vi "from string 2.0.vi"(8 "error in (no error)":errorcluster, 10 "data":string, 11 "PID Module configuration in":refnum<class "PID Module configuration.lvclass">) -> (0 "error out":errorcluster, 3 "PID Module configuration out":refnum<class "PID Module configuration.lvclass">)   [LabVIEW 2015, in "PID Module configuration.lvclass"]
uses:
  PID Module configuration.lvclass
  <vilib>/NI/Tag Bus Module Framework/channel/TBM channel.lvclass
  Line.ctl
  PID Module configuration.lvclass/PID Module configuration.ctl
  <vilib>/NI/Configuration Framework/serializable configuration/NISE_CEF_serializable configuration.lvclass
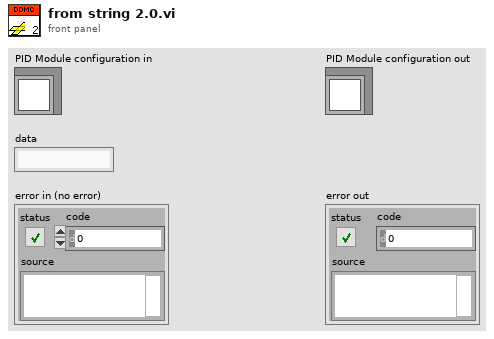
[diagram p1: front panel]
types:
  T1 = typedef "PID Module configuration.lvclass/Line.ctl" = cluster{"PID ID":string, "Setpoint":refnum<class "TBM channel.lvclass">, "Variable":refnum<class "TBM channel.lvclass">, "Output":refnum<class "TBM channel.lvclass">, "Output High":refnum<class "TBM channel.lvclass">, "Output Low":refnum<class "TBM channel.lvclass">, "P":refnum<class "TBM channel.lvclass">, "I":refnum<class "TBM channel.lvclass">, "D":refnum<class "TBM channel.lvclass">}
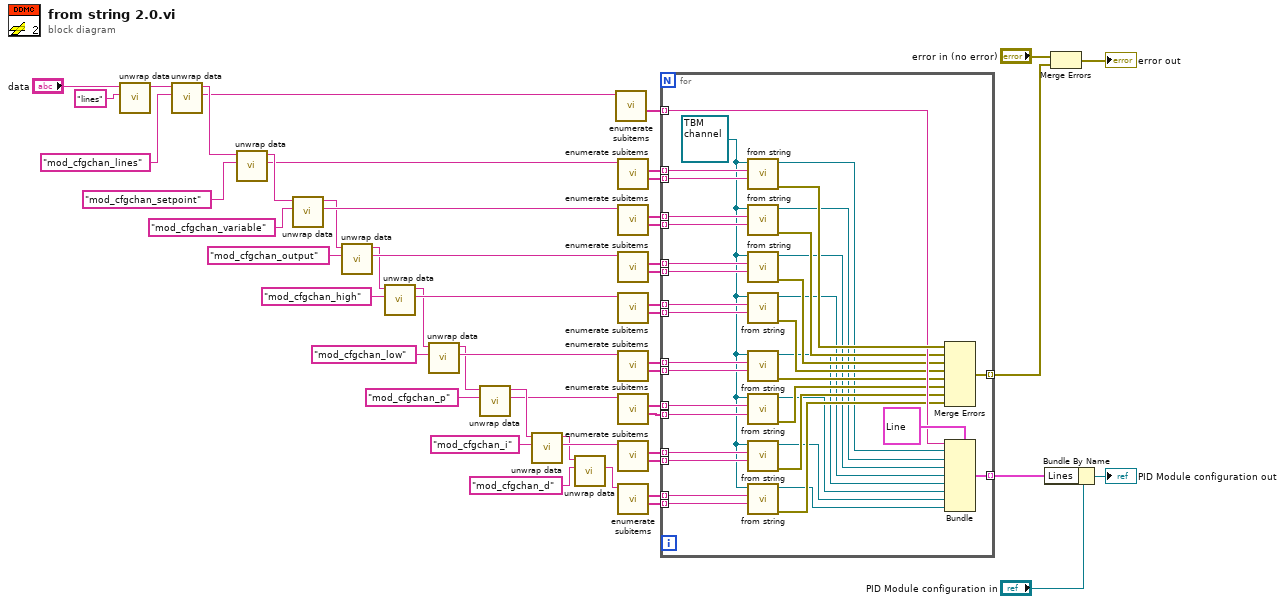
[diagram p0: block diagram]
diagram:
  n1 = call <vilib>:"unwrap data.vi"("identifier"="lines" ("additional identifier"), "data to unwrap"="data") -> ("remaining string"=w49:string)  [unwired: 8 in, 1 out]
  n2 = call <vilib>:"unwrap data.vi"("identifier"="mod_cfgchan_lines", "data to unwrap"=w49) -> ("unwrapped data"=w18:string, "remaining string"=w37:string)  [unwired: 8 in]
  n3 = call <vilib>:"unwrap data.vi"("identifier"="mod_cfgchan_setpoint", "data to unwrap"=w37) -> ("unwrapped data"=w17:string, "remaining string"=w36:string)  [unwired: 8 in]
  n4 = call <vilib>:"unwrap data.vi"("identifier"="mod_cfgchan_variable", "data to unwrap"=w36) -> ("unwrapped data"=w44:string, "remaining string"=w35:string)  [unwired: 8 in]
  n5 = call <vilib>:"unwrap data.vi"("identifier"="mod_cfgchan_output", "data to unwrap"=w35) -> ("unwrapped data"=w43:string, "remaining string"=w34:string)  [unwired: 8 in]
  n6 = call <vilib>:"unwrap data.vi"("identifier"="mod_cfgchan_high", "data to unwrap"=w34) -> ("unwrapped data"=w42:string, "remaining string"=w33:string)  [unwired: 8 in]
  n7 = call <vilib>:"unwrap data.vi"("identifier"="mod_cfgchan_low", "data to unwrap"=w33) -> ("unwrapped data"=w41:string, "remaining string"=w32:string)  [unwired: 8 in]
  n8 = call <vilib>:"unwrap data.vi"("identifier"="mod_cfgchan_p", "data to unwrap"=w32) -> ("unwrapped data"=w22:string, "remaining string"=w31:string)  [unwired: 8 in]
  n9 = call <vilib>:"unwrap data.vi"("identifier"="mod_cfgchan_i", "data to unwrap"=w31) -> ("unwrapped data"=w40:string, "remaining string"=w30:string)  [unwired: 8 in]
  n10 = call <vilib>:"unwrap data.vi"("identifier"="mod_cfgchan_d", "data to unwrap"=w30) -> ("unwrapped data"=w21:string)  [unwired: 8 in, 1 out]
  n11 = call <vilib>:"enumerate subitems.vi"("data to enumerate"=w18) -> ("associated data"=w16:string[])  [unwired: 8 in, 2 out]
  n12 = call <vilib>:"enumerate subitems.vi"("data to enumerate"=w17) -> ("associated data"=w51:string[], "discovered subitems"=w50:string[])  [unwired: 8 in, 1 out]
  n13 = call <vilib>:"enumerate subitems.vi"("data to enumerate"=w44) -> ("associated data"=w14:string[], "discovered subitems"=w15:string[])  [unwired: 8 in, 1 out]
  n14 = call <vilib>:"enumerate subitems.vi"("data to enumerate"=w43) -> ("associated data"=w12:string[], "discovered subitems"=w13:string[])  [unwired: 8 in, 1 out]
  n15 = call <vilib>:"enumerate subitems.vi"("data to enumerate"=w42) -> ("associated data"=w10:string[], "discovered subitems"=w11:string[])  [unwired: 8 in, 1 out]
  n16 = call <vilib>:"enumerate subitems.vi"("data to enumerate"=w41) -> ("associated data"=w8:string[], "discovered subitems"=w9:string[])  [unwired: 8 in, 1 out]
  n17 = call <vilib>:"enumerate subitems.vi"("data to enumerate"=w22) -> ("associated data"=w6:string[], "discovered subitems"=w7:string[])  [unwired: 8 in, 1 out]
  n18 = call <vilib>:"enumerate subitems.vi"("data to enumerate"=w40) -> ("associated data"=w4:string[], "discovered subitems"=w5:string[])  [unwired: 8 in, 1 out]
  n19 = call <vilib>:"enumerate subitems.vi"("data to enumerate"=w21) -> ("associated data"=w2:string[], "discovered subitems"=w3:string[])  [unwired: 8 in, 1 out]
  n20 = for {
    tunnel: w50 -> [w89] mode=indexing
    tunnel: w51 -> [w88] mode=indexing
    tunnel: [w86] -> w52 mode=indexing
    tunnel: [w85] -> w19 mode=indexing
    tunnel: w16 -> [w83] mode=indexing
    tunnel: w15 -> [w82] mode=indexing
    tunnel: w14 -> [w81] mode=indexing
    tunnel: w13 -> [w80] mode=indexing
    tunnel: w12 -> [w79] mode=indexing
    tunnel: w11 -> [w78] mode=indexing
    tunnel: w10 -> [w77] mode=indexing
    tunnel: w9 -> [w76] mode=indexing
    tunnel: w8 -> [w75] mode=indexing
    tunnel: w7 -> [w74] mode=indexing
    tunnel: w6 -> [w73] mode=indexing
    tunnel: w5 -> [w72] mode=indexing
    tunnel: w4 -> [w71] mode=indexing
    tunnel: w3 -> [w70] mode=indexing
    tunnel: w2 -> [w69] mode=indexing
    w61 = refnum<class "TBM channel.lvclass"> refnum ("channel in")
    n21 = call-dynamic "from string.vi"("channel data"=w88, "identifier"=w89, "channel in"=w61) -> ("error out"=w84:errorcluster, "channel out"=w60:refnum<class "TBM channel.lvclass">)  [unwired: 7 in]
    n22 = call-dynamic "from string.vi"("channel data"=w81, "identifier"=w82, "channel in"=w61) -> ("error out"=w68:errorcluster, "channel out"=w59:refnum<class "TBM channel.lvclass">)  [unwired: 7 in]
    n23 = call-dynamic "from string.vi"("channel data"=w79, "identifier"=w80, "channel in"=w61) -> ("error out"=w67:errorcluster, "channel out"=w58:refnum<class "TBM channel.lvclass">)  [unwired: 7 in]
    n24 = call-dynamic "from string.vi"("channel data"=w77, "identifier"=w78, "channel in"=w61) -> ("error out"=w66:errorcluster, "channel out"=w57:refnum<class "TBM channel.lvclass">)  [unwired: 7 in]
    n25 = call-dynamic "from string.vi"("channel data"=w75, "identifier"=w76, "channel in"=w61) -> ("error out"=w65:errorcluster, "channel out"=w56:refnum<class "TBM channel.lvclass">)  [unwired: 7 in]
    n26 = call-dynamic "from string.vi"("channel data"=w73, "identifier"=w74, "channel in"=w61) -> ("error out"=w64:errorcluster, "channel out"=w55:refnum<class "TBM channel.lvclass">)  [unwired: 7 in]
    n27 = call-dynamic "from string.vi"("channel data"=w71, "identifier"=w72, "channel in"=w61) -> ("error out"=w63:errorcluster, "channel out"=w54:refnum<class "TBM channel.lvclass">)  [unwired: 7 in]
    n28 = call-dynamic "from string.vi"("channel data"=w69, "identifier"=w70, "channel in"=w61) -> ("error out"=w62:errorcluster, "channel out"=w53:refnum<class "TBM channel.lvclass">)  [unwired: 7 in]
    n29 = Merge Errors(w84, w68, w67, w66, w65, w64, w63, w62) -> (w85:errorcluster)
    n30 = Bundle(cluster=T1 {"PID ID"="", "Setpoint"=refnum, "Variable"=refnum, "Output"=refnum, "Output High"=refnum, "Output Low"=refnum, "P"=refnum, "I"=refnum, "D"=refnum} ("Line"), "PID ID"=w83, "Setpoint"=w60, "Variable"=w59, "Output"=w58, "Output High"=w57, "Output Low"=w56, "P"=w55, "I"=w54, "D"=w53) -> (w86:T1)
  }
  n31 = Bundle By Name(cluster="PID Module configuration in", "Lines"=w52) -> (→"PID Module configuration out":refnum<class "PID Module configuration.lvclass">)
  n32 = Merge Errors("error in (no error)", w19) -> (→"error out":errorcluster)
